vi "Driver Lists.vi"(11 "error in (no error)":errorcluster) -> (15 "error out":errorcluster)   [LabVIEW 2021, in "Converter.lvlib"]
uses:
  Converter.lvlib
  <vilib>/Utility/traverseref.llb/TRef TravTarget.ctl
  <vilib>/Utility/traverseref.llb/VI Scripting - Traverse.lvlib
  Converter Reusables/Converter Reusables.lvlib
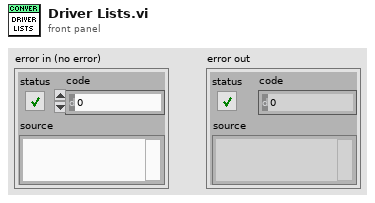
[diagram p1: front panel]
types:
  T1 = typedef "TRef TravTarget.ctl" = enum16{"FP", "BD", "Other"}
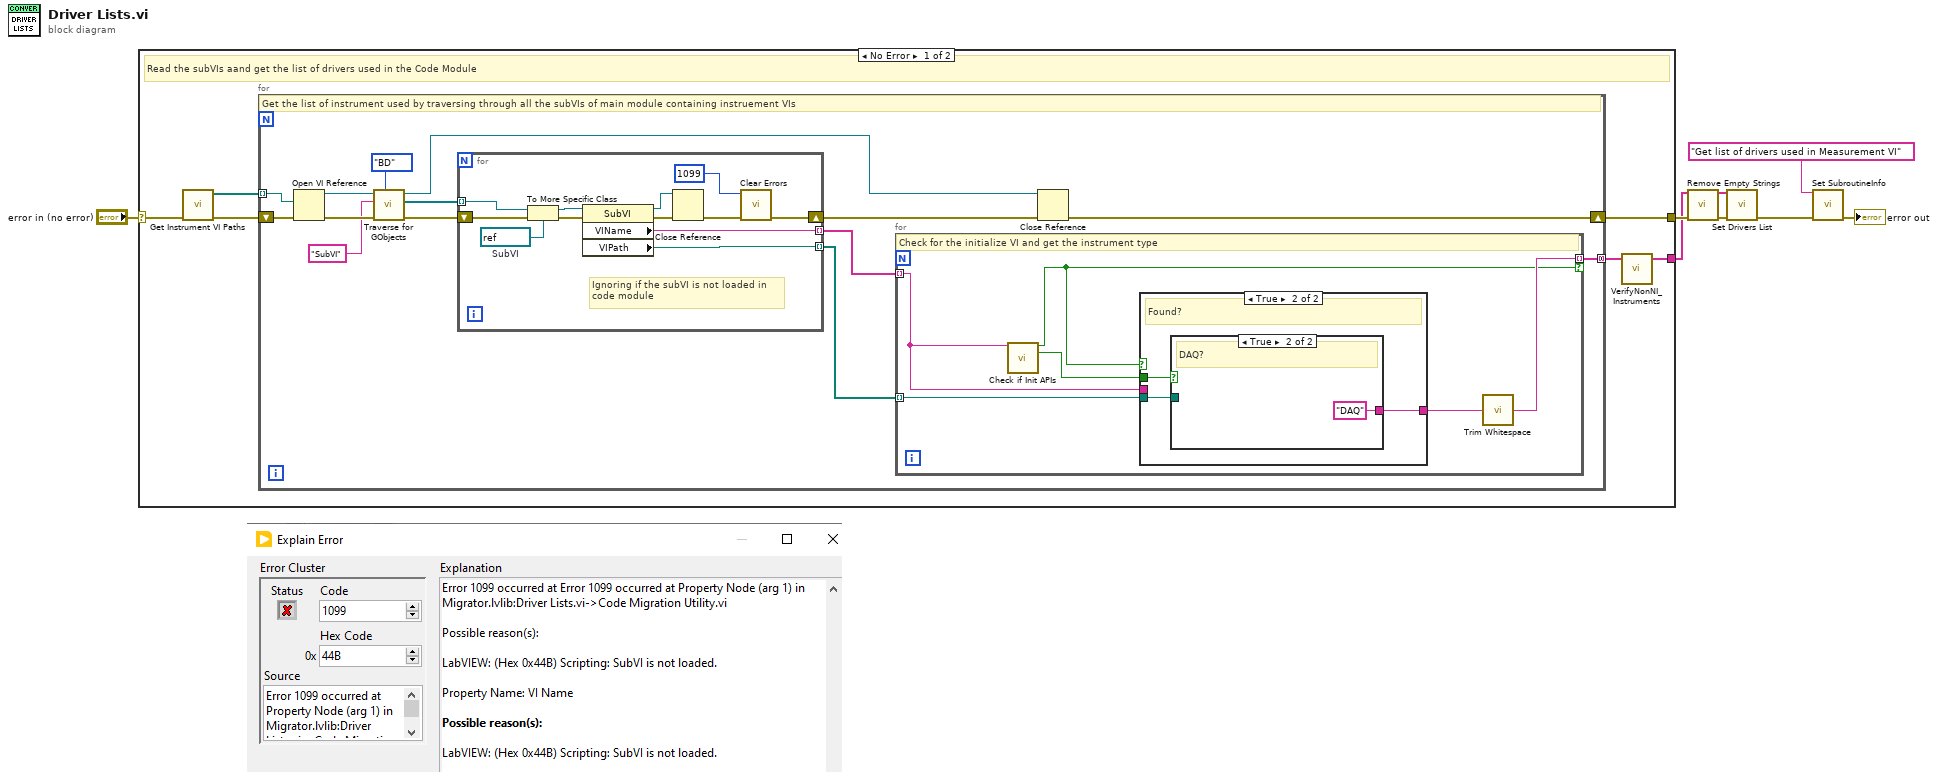
[diagram p0: block diagram]
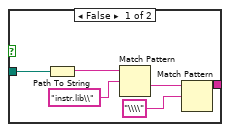
[diagram p3: hidden frame]
diagram:
  n1 = case shown="No Error" "error in (no error)" {
    selector: "error in (no error)" -> [w12 w56]
    tunnel: [w8 w56] -> w6
    tunnel: [w9 _] -> w2
    frame No Error {
      # "Read the subVIs aand get the list of drivers used in the Code Module"
      n2 = call "Get Instrument VI Paths.vi"("error in (no error)"=w12) -> ("error out"=w11:errorcluster, "Instr VI Paths[]"=w13:path[])  [unwired: 9 in]
      n3 = for {
        tunnel: w13 -> [w22] mode=indexing
        tunnel: [w18] -> w10 mode=concatenating
        shift-right: [w16] -> w8
        shift-left: w11 -> [w21]
        # "Get the list of instrument used by traversing through all the subVIs of main module containing instruement VIs"
        n4 = Open VI Reference(vi path=w22, error in (no error)=w21) -> (vi reference=w17:refnum<vi>, error out=w25:errorcluster)  [unwired: 4 in]
        n5 = call <vilib>:"Traverse for GObjects.vi"("Traverse Target"=TRef_TravTarget."BD", "error in (no error)"=w25, "Class Name"="SubVI", "VI Refnum"=w17) -> ("error out"=w27:errorcluster, "References"=w26:refnum<vi>[], "dup VI Refnum"=w14:refnum<vi>)  [unwired: 4 in, 1 out]
        n6 = for {
          tunnel: w26 -> [w54] mode=indexing
          tunnel: [w50] -> w20 mode=indexing
          tunnel: [w49] -> w19 mode=indexing
          shift-right: [w45] -> w15
          shift-left: w27 -> [w53]
          w55 = refnum<vi> refnum  # SubVI
          # "Ignoring if the subVI is not loaded in\ncode module"
          n7 = To More Specific Class(target class=w55, reference=w54, error in=w53) -> (specific class reference=w52:refnum<vi>, error out=w51:errorcluster)
          n8 = property class="SubVI"(reference=w52, error in=w51) -> (reference out=w48:refnum<vi>, error out=w47:errorcluster, "VIName"=w50:string, "VIPath"=w49:path)
          n9 = Close Reference(reference=w48, error in (no error)=w47) -> (error out=w46:errorcluster)
          n10 = call <vilib>:"Clear Errors.vi"("error in (no error)"=w46, "specific error code to clear (0: all)"=1099) -> ("error out"=w45:errorcluster)  [unwired: 4 in, 1 out]
        }
        n11 = for {
          tunnel: w20 -> [w29] mode=indexing
          tunnel: w19 -> [w33] mode=indexing
          tunnel: [w32] -> w18 mode=indexing if=w30
          # "Check for the initialize VI and get the instrument type"
          n12 = call "Check if Init APIs.vi"("VIName"=w29) -> ("Instrument Driver Found?"=w30:bool, "DAQ?"=w28:bool)  [unwired: 13 in]
          n13 = case shown="True" w30 {
            tunnel: w33 -> [_ w36]
            tunnel: [_ w35] -> w31
            tunnel: w29 -> [_ _]
            tunnel: w28 -> [_ w34]
            frame False {
            }
            frame True {
              # "Found?"
              n14 = case shown="True" w34 {
                tunnel: w36 -> [w38 _]
                tunnel: [w37 "DAQ"] -> w35
                frame False {
                  n15 = Path To String(path=w38) -> (string=w39:string)
                  n16 = Match Pattern(string=w39, regular expression="instr.lib\\") -> (after substring=w41:string)  [unwired: 1 in, 3 out]
                  n17 = Match Pattern(string=w41, regular expression="\\\\") -> (before substring=w37:string)  [unwired: 1 in, 3 out]
                }
                frame True {
                  # "DAQ?"
                }
              }
            }
          }
          n18 = call <vilib>:"Trim Whitespace.vi"("string"=w31) -> ("trimmed string"=w32:string)  [unwired: 1 in]
        }
        n19 = Close Reference(reference=w14, error in (no error)=w15) -> (error out=w16:errorcluster)
      }
      n20 = call "VerifyNonNI_Instruments.vi"("Instrument Types In"=w10) -> ("Instrument Types Out"=w9:string[])  [unwired: 4 in]
    }
    frame Error {
    }
  }
  n21 = call "Remove Empty Strings.vi"("Instrument Types Out in"=w2) -> ("Instrument Types Out out"=w1:string[])  [unwired: 14 in]
  n22 = call "Set Drivers List.vi"("Name"=w1, "error in (no error)"=w6) -> ("error out"=w5:errorcluster)  [unwired: 13 in]
  n23 = call "Set SubroutineInfo.vi"("Subroutine In"="Get list of drivers used in Measurement VI", "error in (no error)"=w5) -> ("error out"=→"error out":errorcluster)  [unwired: 13 in]
